vi "Test Find Node.vi"(8 "error in (no error)":errorcluster) -> (0 "error out":errorcluster)   [LabVIEW 2017, in "Unit Tests.lvlib"]
uses:
  Unit Tests.lvlib
  source/Browser Core/Server Classes/Base Tree/Base Tree.lvclass
  source/Browser Core/Node Classes/Generic Node/Generic Node.lvclass
  source/Browser Core/Server Classes/Base Tree/Base Tree.lvclass/Base Tree.ctl
  <vilib>/addons/_JKI Toolkits/Caraya/classes/Test/Test.lvclass
  <vilib>/addons/_JKI Toolkits/Caraya/classes/Assert/Assert.lvclass
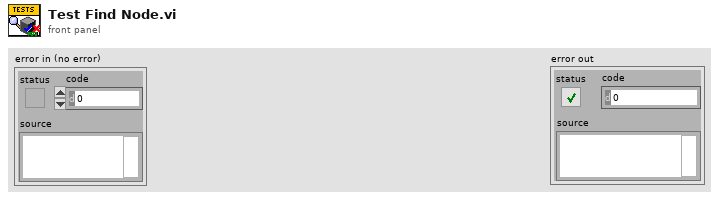
[diagram p1: front panel]
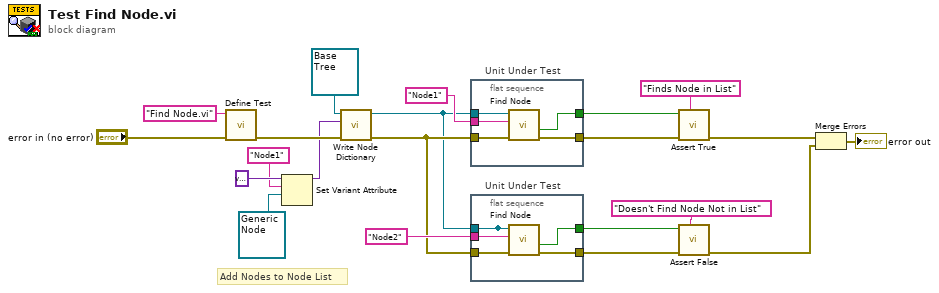
[diagram p0: block diagram]
diagram:
  # "Add Nodes to Node List"
  n1 = call <vilib>:"Define Test.vi"("error in (no error)"="error in (no error)", "Label (VI Title)"="Find Node.vi") -> ("error out"=w5:errorcluster)  [unwired: 9 in]
  n2 = Set Variant Attribute(Variant=variant ("Node Dictionary"), name="Node1" ("UID"), value=refnum<class "Generic Node.lvclass"> refnum ("Node")) -> (Variant out=w2:variant)  [unwired: 1 in, 2 out]
  n3 = call "Write Node Dictionary.vi"("error in (no error)"=w5, "Node Dictionary"=w2, "Base Tree in"=refnum<class "Base Tree.lvclass"> refnum) -> ("error out"=w4:errorcluster, "Base Tree out"=w3:refnum<class "Base Tree.lvclass">)  [unwired: 7 in]
  n4 = flat-sequence "Unit Under Test" {
    tunnel: w4 -> [w26]
    tunnel: w3 -> [w25]
    tunnel: "Node1" ("UID") -> [w24]
    tunnel: [w23] -> w18
    tunnel: [w22] -> w14
    frame #0 {
      n5 = call-dynamic "Find Node.vi"("error in (no error)"=w26, "UID"=w24, "Base Tree in"=w25) -> ("error out"=w23:errorcluster, "Found?"=w22:bool)  [unwired: 5 in, 2 out]
    }
  }
  n6 = flat-sequence "Unit Under Test" {
    tunnel: w4 -> [w31]
    tunnel: [w28] -> _
    tunnel: "Node2" ("UID") -> [w30]
    tunnel: [w29] -> w16
    tunnel: w3 -> [w28]
    tunnel: [w27] -> w15
    frame #0 {
      n7 = call-dynamic "Find Node.vi"("error in (no error)"=w31, "UID"=w30, "Base Tree in"=w28) -> ("error out"=w29:errorcluster, "Found?"=w27:bool)  [unwired: 5 in, 2 out]
    }
  }
  n8 = call <vilib>:"Assert True.vi"("Label"="Finds Node in List", "error in (no error)"=w18, "True?"=w14) -> ("error out"=w11:errorcluster)  [unwired: 8 in]
  n9 = call <vilib>:"Assert False.vi"("Label"="Doesn't Find Node Not in List", "error in (no error)"=w16, "False?"=w15) -> ("error out"=w10:errorcluster)  [unwired: 8 in]
  n10 = Merge Errors(w11, w10) -> (→"error out":errorcluster)
